vi "ForwardPropagation.vi"(10 "Array in":dbl[](array[numeric]), 11 "Array 3":cluster{"A - B":T1}[](array[cluster])) -> (3 "Array out":cluster{dbl[]}[](array[cluster]))   [LabVIEW 2016]
uses:
  <vilib>/Analysis/Matrix/Datatypes/RealMatrix.ctl
  <vilib>/Analysis/baseanly.llb/A x Vector.vi
  <vilib>/Analysis/NI_AALBase.lvlib
  <vilib>/Analysis/Matrix/NI_Matrix.lvlib
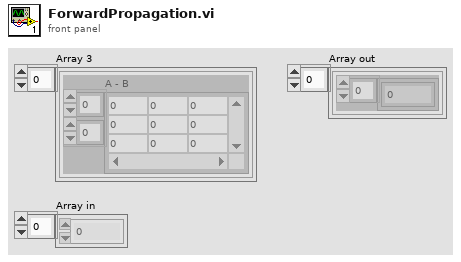
[diagram p1: front panel]
types:
  T1 = typedef "NI_Matrix.lvlib/RealMatrix.ctl" = dbl[][]
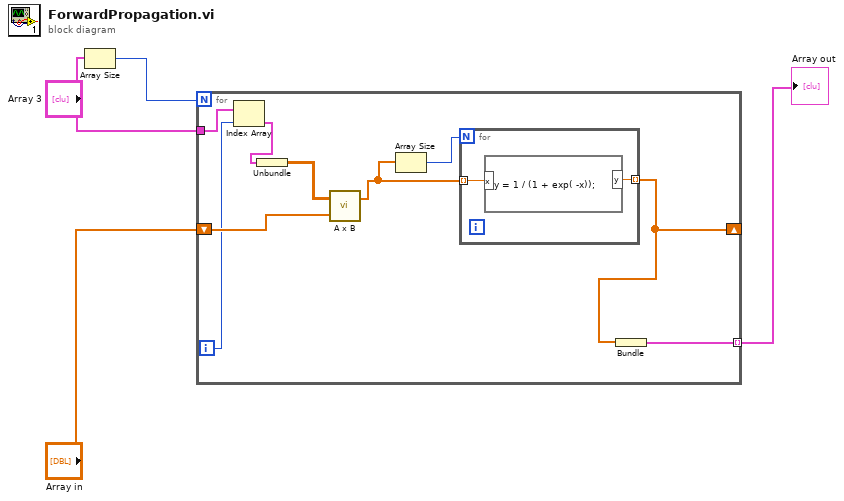
[diagram p0: block diagram]
diagram:
  n1 = Array Size(array="Array 3") -> (size(s)=w1:i32)
  n2 = for {
    N: w1 -> [_]
    tunnel: "Array 3" -> [w7]
    shift-right: [w10] -> _
    shift-left: "Array in" -> [w11]
    tunnel: [w5] -> w4 mode=indexing
    i -> [w8]
    n3 = Index Array(array=w7, index=w8) -> (element=w6:cluster{"A - B":T1})
    n4 = Unbundle(w6) -> ("A - B"=w13:T1)
    n5 = call-poly <vilib>:"A x B.vi"("Vector"=w11, "A"=w13) -> ("A x Vector"=w9:dbl[])  [unwired: 1 out]
    n6 = Array Size(array=w9) -> (size(s)=w12:i32)
    n7 = for {
      N: w12 -> [_]
      tunnel: w9 -> [w15] mode=indexing
      tunnel: [w14] -> w10 mode=indexing
      n8 = formula code="y = 1 / (1 + exp( -x));"("x"=w15) -> ("y"=w14:dbl)
    }
    n9 = Bundle(w10) -> (w5:cluster{dbl[]})  [unwired: 1 in]
  }
  "Array out" <- w4
